vi "Der_ReLU.vi"(1 "A_l":T1) -> (0 "g'(Z)":T1)   [LabVIEW 2016]
uses:
  <vilib>/Analysis/Matrix/Datatypes/RealMatrix.ctl
  <vilib>/Analysis/Matrix/Numeric/Conversions/Matrix To Array - RM.vi
  <vilib>/Analysis/Matrix/Numeric/Conversions/Array To Matrix - RA2.vi
  <vilib>/Analysis/Matrix/NI_Matrix.lvlib
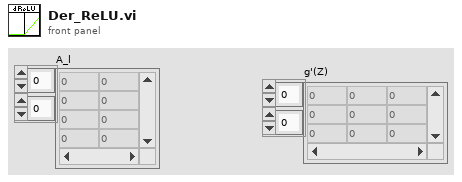
[diagram p1: front panel]
types:
  T1 = typedef "NI_Matrix.lvlib/RealMatrix.ctl" = dbl[][]
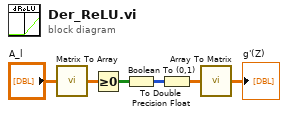
[diagram p0: block diagram]
diagram:
  n1 = call-poly <vilib>:"Matrix To Array.vi"("Real Matrix"="A_l") -> ("Real 2D Array"=w5:dbl[][])
  n2 = Greater Or Equal To 0?(x=w5) -> (x >= 0?=w4:bool[][])
  n3 = Boolean To (0,1)(Boolean=w4) -> (0, 1=w3:i16[][])
  n4 = To Double Precision Float(number=w3) -> (double precision float=w2:dbl[][])
  n5 = call-poly <vilib>:"Array To Matrix.vi"("Real 2D Array"=w2) -> ("Real Matrix"=→"g'(Z)":T1)
